vi "Set_Read_IP_Addresses.vi"(3 "New IP Address":string) -> (1 "IP Addresses":string[](array[string]))   [LabVIEW 2009]
uses:
  <vilib>/Utility/config.llb/Read Key (String).vi
  <vilib>/Utility/config.llb/Write Key (String).vi
  <vilib>/Utility/config.llb/NI_LVConfig.lvlib
panel:
  out "List of IP":string
  # "This LabVIEW item is deprecated.\n\nIt is believed to be unused and will be removed in a future version of SRV."
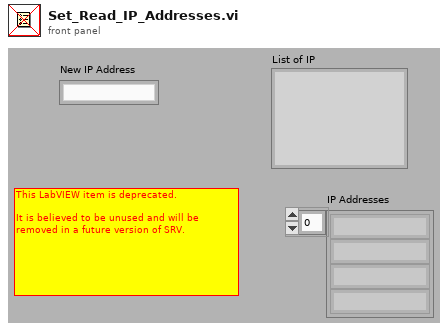
[diagram p1: front panel]
types:
  T1 = typedef "NI_LVConfig.lvlib/Config Data RefNum.ctl" = refnum<k1>
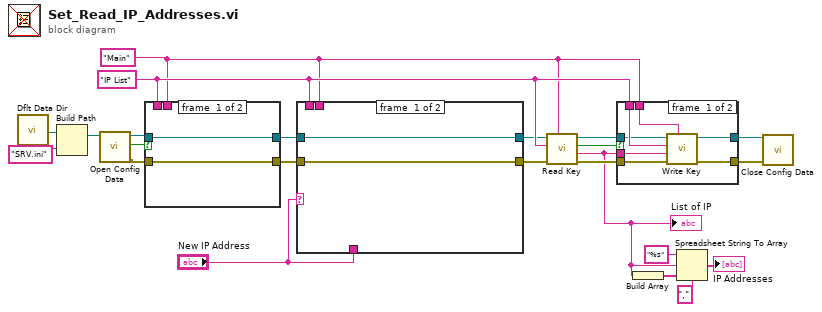
[diagram p0: block diagram]
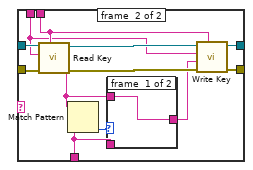
[diagram p2: hidden frame]
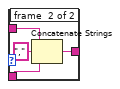
[diagram p3: hidden frame]
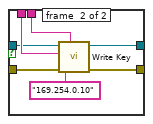
[diagram p4: hidden frame]
diagram:
  w4 = "Main" ("section")
  w5 = "IP List" ("key")
  n1 = call <vilib>:"Dflt Data Dir.vi"() -> ("App:Default Data Directory"=w23:path)
  n2 = Build Path(base path=w23, name or relative path="SRV.ini") -> (appended path=w21:path)
  n3 = call <vilib>:"Open Config Data.vi"("configuration file path"=w21) -> ("error out"=w13:errorcluster, "file created?"=w15:bool, "refnum"=w14:T1)  [unwired: 8 in]
  n4 = case shown="True" w15 {
    tunnel: w13 -> [w24 w32]
    tunnel: w5 -> [_ w31]
    tunnel: w4 -> [_ w30]
    tunnel: w14 -> [w25 w29]
    tunnel: [w25 w28] -> w7
    tunnel: [w24 w27] -> w6
    frame #0 {
    }
    frame #1 {
      n5 = call-poly <vilib>:"Write Key.vi"("section"=w30, "error in (no error)"=w32, "value"="169.254.0.10" ("default value"), "key"=w31, "refnum"=w29) -> ("error out"=w27:errorcluster, "refnum out"=w28:T1)  [unwired: 4 in, 1 out]
    }
  }
  n6 = case shown="Default" "New IP Address" {
    tunnel: w6 -> [w33 w44]
    tunnel: w5 -> [_ w39]
    tunnel: w4 -> [_ w41]
    tunnel: w7 -> [w34 w42]
    tunnel: [w34 w46] -> w3
    tunnel: [w33 w45] -> w2
    tunnel: "New IP Address" -> [_ w36]
    frame #0 {
    }
    frame #1 {
      n7 = call-poly <vilib>:"Read Key.vi"("section"=w41, "error in (no error)"=w44, "key"=w39, "refnum"=w42) -> ("error out"=w43:errorcluster, "value"=w37:string, "refnum out"=w40:T1)  [unwired: 4 in, 1 out]
      n8 = Match Pattern(string=w37, regular expression=w36) -> (offset past match=w38:i32)  [unwired: 1 in, 3 out]
      n9 = case shown="-1" w38 {
        tunnel: w37 -> [w47 w51]
        tunnel: w36 -> [_ w50]
        tunnel: [w47 w48] -> w35
        frame #0 {
        }
        frame #1 {
          n10 = Concatenate Strings(w51, "," ("string"), w50) -> (w48:string)
        }
      }
      n11 = call-poly <vilib>:"Write Key.vi"("section"=w41, "error in (no error)"=w43, "value"=w35, "key"=w39, "refnum"=w40) -> ("error out"=w45:errorcluster, "refnum out"=w46:T1)  [unwired: 4 in, 1 out]
    }
  }
  n12 = call-poly <vilib>:"Read Key.vi"("section"=w4, "error in (no error)"=w2, "key"=w5, "refnum"=w3) -> ("error out"=w20:errorcluster, "value"=w10:string, "found?"=w16:bool, "refnum out"=w19:T1)  [unwired: 4 in]
  "List of IP" <- w10
  n13 = case shown="False" w16 {
    tunnel: w20 -> [w58 w59]
    tunnel: w5 -> [w57 _]
    tunnel: w4 -> [w56 _]
    tunnel: w19 -> [w55 w60]
    tunnel: w10 -> [w54 _]
    tunnel: [w53 w60] -> w18
    tunnel: [w52 w59] -> w17
    frame #0 {
      n14 = call-poly <vilib>:"Write Key.vi"("section"=w56, "error in (no error)"=w58, "value"=w54, "key"=w57, "refnum"=w55) -> ("error out"=w52:errorcluster, "refnum out"=w53:T1)  [unwired: 4 in, 1 out]
    }
    frame #1 {
    }
  }
  n15 = Build Array(w10) -> (w9:string[])
  n16 = Spreadsheet String To Array(delimiter (Tab)=",", format string="%s", spreadsheet string=w10, array type (2D Dbl)=w9) -> (array=→"IP Addresses":string[])
  n17 = call <vilib>:"Close Config Data.vi"("error in (no error)"=w17, "refnum"=w18) -> ()  [unwired: 8 in, 2 out]
